vi "RT_Main.vi"() -> ()   [LabVIEW 2018]
doc: "Main VI running on the RT Target."
uses:
  Typedefs/StateDef_Enum.ctl
  <vilib>/Platform/TimedLoop/XDataNode/timing_clust.ctl
  <vilib>/Platform/TimedLoop/XDataNode/nitl_modes.ctl
  <vilib>/Platform/TimedLoop/XDataNode/wakeup.ctl
  <vilib>/FPGAPlugInAG/myRIO-1900/niLvFpga_Open_myRIO-1900.vi
  <vilib>/rvi/interface/common/dynamic/niFpgaDynamicAddResources.vi
  <vilib>/Utility/error.llb/Error Cluster From Error Code.vi
  <vilib>/rvi/errors/niLvFpgaAdjustHostInterfaceError.vi
  <vilib>/FPGAPlugInAG/Dynamic/niLvFpga_Close_Dynamic.vi
  <vilib>/Platform/TimedLoop/XDataNode/XDataNode.xnode
  <vilib>/rvi/interface/nirviOpenFPGA/nirviOpenFPGA.xnode
  FPGA Bitfiles/ScaleReader_FPGATarget_FPGAmain_v3.lvbitx
  <vilib>/rvi/interface/nirviReadWriteControl/nirviReadWriteControl.xnode
  <vilib>/rvi/interface/nirviCloseFPGA/nirviCloseFPGA.xnode
  Components/Timing/Timing.lvlib
  <vilib>/Platform/TimedLoop/XDataNode/XDNodeRunTimeDep.lvlib
  Components/WeightMeas/WeightMeas.lvlib
  <vilib>/rvi/interface/Simulation/niFpgaSimulationCallBeginRW.vi
  NiFpgaLv.dll
panel:
  in  "Pause chart?":bool
  out "Status":string
  in  "System Stop Button":bool
  in  "Loop Timing":enum32{"Algo.", "UI"}(tab)
  out "# Finished\nLate counter":dbl
  in  "Algorithm\nLoop Rate (Hz)":dbl=1000.0 format="%#_4p"
  in  "UI Loop rate (Hz)":dbl=1000.0 format="%#_6p"
  out "Acquired Data":cluster{"Double":dbl, "Double":dbl}(graph)
  out "Load offset \nindicator (kg)":dbl
  in  "Tare Button":bool
  out "Load":dbl format="%.4f"
  # "2.737 Weighing-scale Reader"
  # "Algorithm Loop Timing"
  # "kg"
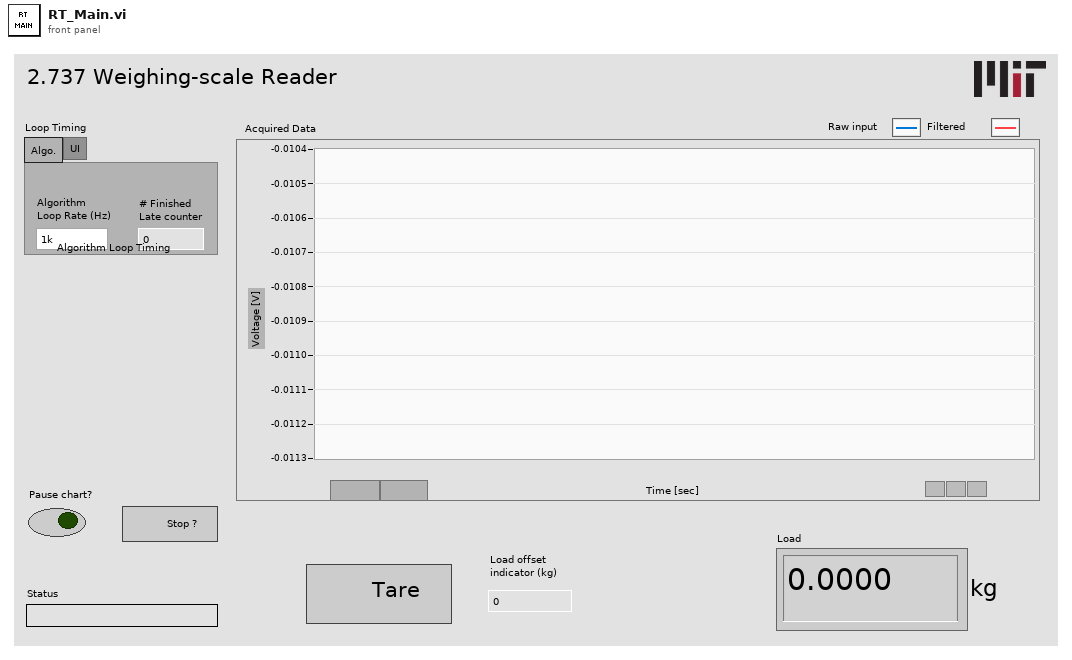
[diagram p1: front panel]
types:
  T1 = typedef "StateDef_Enum.ctl" = enum16{"Initialize", "Wait", "Shutdown"}
  T2 = typedef "XDNodeRunTimeDep.lvlib/timing_clust.ctl" = cluster{"Expected End [f-1]":u64, "Actual End [f-1]":u64, "Finished Late? [f-1]":bool, "Expected End [i-1]":u64, "Actual End [i-1]":u64, "Finished Late? [i-1]":bool, "Expected Start [i]":u64, "Actual Start [i]":u64, "Expected Start [f]":u64, "Actual Start [f]":u64, "Source Name":string, "Structure Name":string, "Period":i64, "Deadline":i64, "Offset":i64, "Start":i64, "Priority":i32, "Timeout":i32, "Mode":T3, "Wakeup Reason":T4, "Error":errorcluster, "Source Type":string, "Secondary Source Type":string, "Global End Time":u64, "Global Start Time":u64, "Frame Duration":u64, "Iteration Duration":u64, "Assigned CPU":i32, "I/O Scan Engine Mode":u32}
  T3 = typedef "XDNodeRunTimeDep.lvlib/nitl_modes.ctl" = enum32{"No Change", "Process missed periods, maintain original phase", "Discard missed periods, maintain original phase", "Process missed periods, ignore original phase", "Discard missed periods, ignore original phase"}
  T4 = typedef "XDNodeRunTimeDep.lvlib/wakeup.ctl" = enum32{"Normal", "Aborted", "Asynchronous wakeup", "Timing source error", "Timed loop error", "Timeout"}
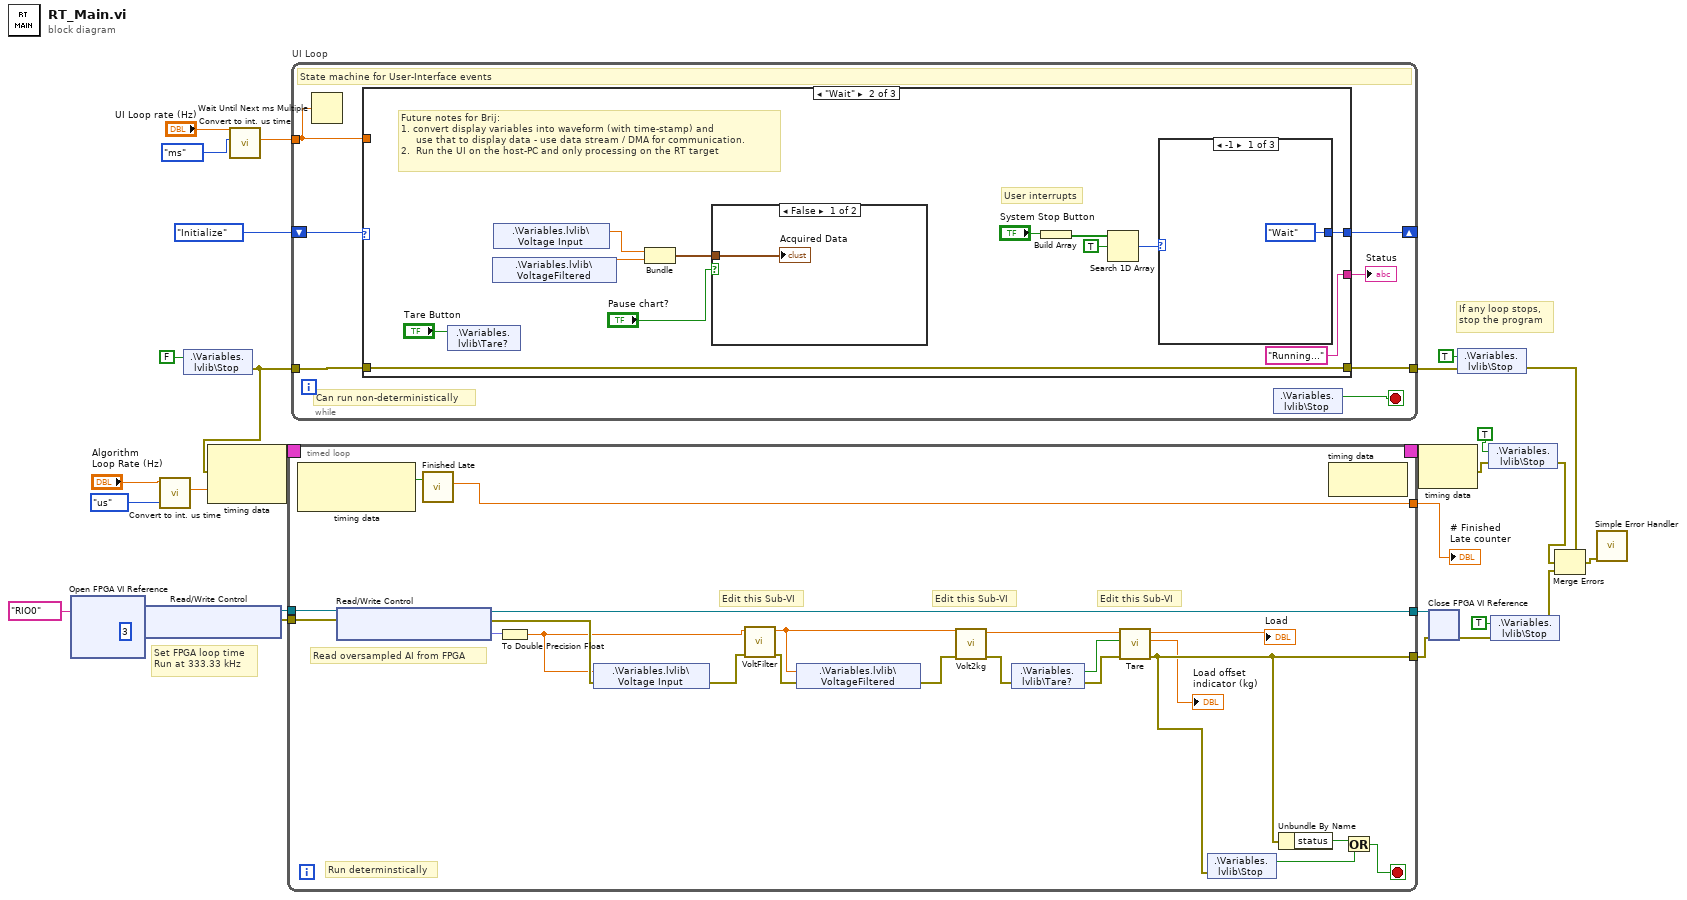
[diagram p0: block diagram]
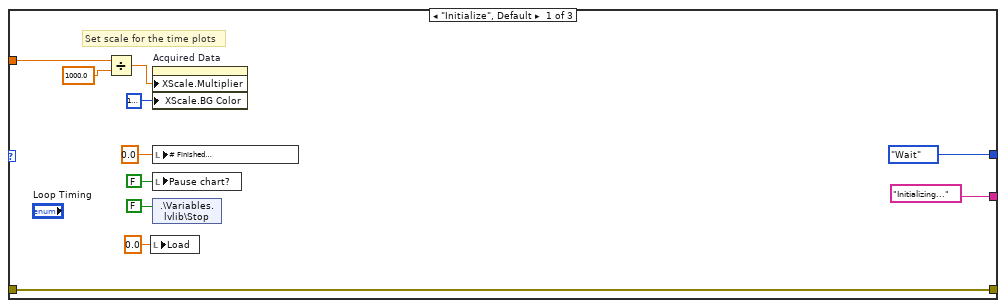
[diagram p2: hidden frame]
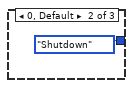
[diagram p4: hidden frame]
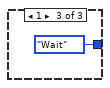
[diagram p5: hidden frame]
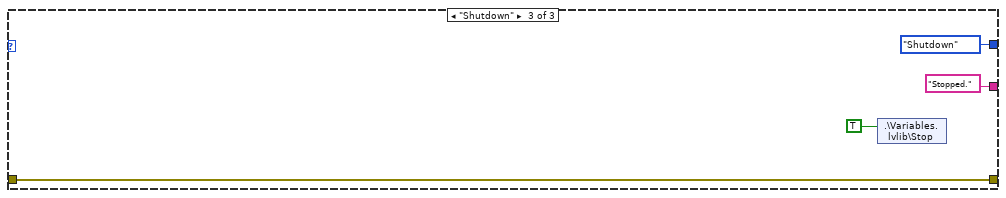
[diagram p6: hidden frame]
diagram:
  # "Set FPGA loop time\nRun at 333.33 kHz"
  # "If any loop stops, \nstop the program"
  n1 = xnode "Open FPGA VI Reference"("resource name"=tag "RIO0") -> ("FPGA VI Reference Out"=w5:refnum<k20>, "error out"=w3:errorcluster)  [unwired: 1 in]
  n2 = xnode "Read/Write Control"("FPGA VI Reference In"=w5, "error in"=w3, "Signal I/O loop rate (us)"=u8 3 ("Count(uSec)")) -> ("FPGA VI Reference Out"=w4:refnum<k20>, "error out"=w2:errorcluster)
  n3 = call "Convert to int. us time.vi"("Int. Time Unit"=enum16{"sec", "us", "ms"}."us", "Sample rate (Hz)"="Algorithm\nLoop Rate (Hz)") -> ("Int.  time [unit]"=w21:dbl)  [unwired: 7 in, 2 out]
  n4 = shared-variable ".\\Variables.lvlib\\Stop"(FALSE ("Stop")) -> (error out=w16:errorcluster)  [unwired: 1 in]
  n5 = node-c288(w16, w21) -> (w25:T2)
  n6 = call "Convert to int. us time.vi"("Int. Time Unit"=enum16{"sec", "us", "ms"}."ms", "Sample rate (Hz)"="UI Loop rate (Hz)") -> ("Int.  time [unit]"=w27:dbl)  [unwired: 7 in, 2 out]
  n7 = timed-loop {
    timing: w25 -> [_]
    timing-out: [_] -> w24
    tunnel: [w51] -> w20
    tunnel: w4 -> [w50]
    tunnel: [w49] -> w19
    tunnel: [w41] -> w17
    tunnel: w2 -> [w34]
    stop <- w43 stop-if-true
    # "Read oversampled AI from FPGA"
    # "Edit this Sub-VI"
    # "Run determinstically"
    # "Edit this Sub-VI"
    # "Edit this Sub-VI"
    n8 = node-c288() -> (w52:bool)  [unwired: 1 in, 1 out]
    n9 = xnode "Read/Write Control"("FPGA VI Reference In"=w50, "error in"=w34) -> ("FPGA VI Reference Out"=w49:refnum<k20>, "error out"=w32:errorcluster, "ConnectorC/AI0 [Filtered]"=w33:fxp<+/-,22,5>)
    n10 = call "Finished Late.vi"("Finished \nLate?"=w52) -> ("# Finished\nLate counter"=w51:dbl)  [unwired: 8 in, 2 out]
    n11 = To Double Precision Float(number=w33) -> (double precision float=w31:dbl)
    n12 = shared-variable ".\\Variables.lvlib\\Voltage Input"(w31, error in=w32) -> (error out=w46:errorcluster)
    n13 = call "VoltFilter.vi"("error in (no error)"=w46, "Voltage In [V]"=w31) -> ("error out"=w45:errorcluster, "Voltage Out [V]"=w48:dbl)  [unwired: 8 in]
    n14 = shared-variable ".\\Variables.lvlib\\VoltageFiltered"(w48, error in=w45) -> (error out=w47:errorcluster)
    n15 = call "Volt2kg.vi"("error in (no error)"=w47, "Voltage In [V]"=w48) -> ("error out"=w37:errorcluster, "Weight Out [kg]"=w40:dbl)  [unwired: 8 in]
    n16 = shared-variable ".\\Variables.lvlib\\Tare?"(error in=w37) -> (w35:bool, error out=w36:errorcluster)
    n17 = call "Tare.vi"("error in (no error)"=w36, "Tare?"=w35, "Uncorrected Load In [kg]"=w40) -> ("error out"=w41:errorcluster, "Load offset [kg]"=→"Load offset \nindicator (kg)":dbl, "Corrected load out [kg]"=→"Load":dbl)  [unwired: 6 in]
    n18 = shared-variable ".\\Variables.lvlib\\Stop"(error in=w41) -> (w42:bool)  [unwired: 1 out]
    n19 = Unbundle By Name(w41) -> ("status"=w44:bool)
    n20 = node-c288() -> ()  [unwired: 1 in, 1 out]
    n21 = Or(x=w44, y=w42) -> (x .or. y?=w43:bool)
  }
  "# Finished\nLate counter" <- w20
  n22 = while "UI Loop" {
    shift-right: [w61] -> _
    shift-left: StateDef_Enum."Initialize" ("State defining Enum") -> [w62]
    tunnel: w16 -> [w60]
    tunnel: [w59] -> w11
    tunnel: w27 -> [w56]
    stop <- w58 stop-if-true
    # "Can run non-deterministically"
    # "State machine for User-Interface events"
    n23 = Wait Until Next ms Multiple(millisecond multiple=w56) -> ()  [unwired: 1 out]
    n24 = case shown="\"Wait\"" w62 {
      tunnel: [StateDef_Enum."Wait" ("State defining Enum") w83 StateDef_Enum."Shutdown" ("State defining Enum")] -> w61
      tunnel: w60 -> [w71 w81 w93]
      tunnel: [w71 w81 w93] -> w59
      tunnel: ["Initializing..." ("Status") "Running..." ("Status") "Stopped." ("Status")] -> w57
      tunnel: w56 -> [w64 _ _]
      frame "Initialize", Default {
        # "Set scale for the time plots"
        n25 = Divide(x=w64, y=1000.0) -> (x/y=w65:dbl)
        n26 = local write "Load"(0.0 ("Load")) -> ()
        n27 = property on="Acquired Data" class="WFChart (strict)"("XScale.Multiplier"=w65, "XScale.BG Color"=u32 16777216) -> ()  [unwired: 2 in, 2 out]
        n28 = local write "# Finished\nLate counter"(0.0 ("# Finished\nLate counter")) -> ()
        n29 = local write "Pause chart?"(FALSE ("Pause chart?")) -> ()
        n30 = shared-variable ".\\Variables.lvlib\\Stop"(FALSE ("Stop?")) -> ()  [unwired: 1 in, 1 out]
      }
      frame "Wait" {
        # "User interrupts"
        # "Future notes for Brij:\n1. convert display variables into waveform (with time-stamp) and\n     use that to display data - use data stream / DMA for communication.\n2.  Run the UI on the host-PC and only processing on the RT target"
        n31 = shared-variable ".\\Variables.lvlib\\Tare?"("Tare Button") -> ()  [unwired: 1 in, 1 out]
        n32 = shared-variable ".\\Variables.lvlib\\VoltageFiltered"() -> (w76:dbl)  [unwired: 1 in, 1 out]
        n33 = shared-variable ".\\Variables.lvlib\\Voltage Input"() -> (w77:dbl)  [unwired: 1 in, 1 out]
        n34 = Bundle("Double"=w77, "Double"=w76) -> (w75:cluster{"Double":dbl, "Double":dbl})  [unwired: 1 in]
        n35 = case shown="False" "Pause chart?" {
          tunnel: w75 -> [w86 _]
          frame False {
            "Acquired Data" <- w86
          }
          frame True {
            # "If pause chart? is true, \nthen stop plotting for a while"
          }
        }
        n36 = Build Array("System Stop Button") -> (w85:bool[])
        n37 = Search 1D Array(1D array=w85, element=TRUE) -> (index of element=w82:i32)  [unwired: 1 in]
        n38 = case shown="-1" w82 {
          tunnel: [StateDef_Enum."Wait" ("State defining Enum") StateDef_Enum."Shutdown" ("State defining Enum") StateDef_Enum."Wait" ("State defining Enum")] -> w83
          frame -1 {
          }
          frame 0, Default {
          }
          frame 1 {
          }
        }
      }
      frame "Shutdown" {
        n39 = shared-variable ".\\Variables.lvlib\\Stop"(TRUE) -> ()  [unwired: 1 in, 1 out]
      }
    }
    "Status" <- w57
    n40 = shared-variable ".\\Variables.lvlib\\Stop"() -> (w58:bool)  [unwired: 1 in, 1 out]
  }
  n41 = node-c288(w24) -> (w9:errorcluster)
  n42 = xnode "Close FPGA VI Reference"("FPGA VI Reference In"=w19, "error in"=w17) -> ("error out"=w14:errorcluster)
  n43 = shared-variable ".\\Variables.lvlib\\Stop"(TRUE ("Stop?"), error in=w11) -> (error out=w10:errorcluster)
  n44 = shared-variable ".\\Variables.lvlib\\Stop"(TRUE ("Stop"), error in=w9) -> (error out=w8:errorcluster)
  n45 = shared-variable ".\\Variables.lvlib\\Stop"(TRUE ("Stop?"), error in=w14) -> (error out=w13:errorcluster)
  n46 = Merge Errors(w10, w8, w13) -> (w18:errorcluster)
  n47 = call <vilib>:"Simple Error Handler.vi"("error in (no error)"=w18) -> ()  [unwired: 4 in, 5 out]
